vi "test222.vi"() -> ()   [LabVIEW 2014]
uses:
  ProjectLocker/NHMFL/LANL/Libraries/maglab ultrasound -- arkady/cursor winow.ctl
  ProjectLocker/NHMFL/LANL/Libraries/maglab ultrasound -- arkady/cursor window action.ctl
panel:
  in  "cursor bracket: All, data window":T1={"left"=3611.67564952785, "right "=3696.4045104721504, "center"=3654.04008, "window"=84.7288609443, "cursors"=[0, 1, 2], "relative"=1, "absolute"=1, "fixed vertical offset"=0.0, "vertical offset"=0.0, "skew"=0.0, "default window frac"=0.1, "kind"=enum."symmetric", "skew.left"=0.5, "skew.right"=0.5, "Plot ref"=refnum, "wing order"=enum."forw"}
  out "Plot: All":cluster{"all rows":dbl[], "all rows":dbl[]}[](graph)
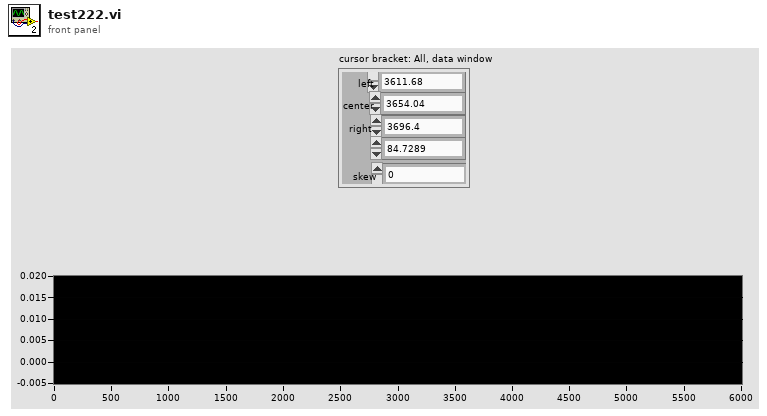
[diagram p1: front panel]
types:
  T1 = typedef "cursor winow.ctl" = cluster{"left":dbl, "right ":dbl, "center":dbl, "window":dbl, "cursors":i32[], "relative":i32, "absolute":i32, "fixed vertical offset":dbl, "vertical offset":dbl, "skew":dbl, "default window frac":dbl, "kind":enum16{"symmetric", "skewed", "fancy"}, "skew.left":dbl, "skew.right":dbl, "Plot ref":refnum<vi>, "wing order":enum16{"forw", "back"}}
  T2 = typedef "cursor window action.ctl" = enum16{"balance", "h. offset change", "cursor moves", "change center", "change window", "init", "check", "reset", "set y to middle", "idle", "-write all Y", "-write left.X", "-write center.X", "-write right.X", "-write all X", "-change center", "-change window", "-change skew", "-read cursor 2", "-read cursor 1", "-read cursor 0", "-read all cursors", "-reset", "-read plot scale", "-set y to middle", "-Q: center.Y is visible", "-Q: window is visible", "-parse center.Y", "-right left from center", "-left move", "-right move", "-set center.Y", "-empty", "-set cursors to default", "-check", "-write center.Y", "-copy cursor 1", "-copy cursor 0", "-copy cursor 2", "move right", "move left", "shrink", "broaden", "skew up", "skew down", "-write plot scale", "zoom X", "change cen&win", "zoom to all data"}
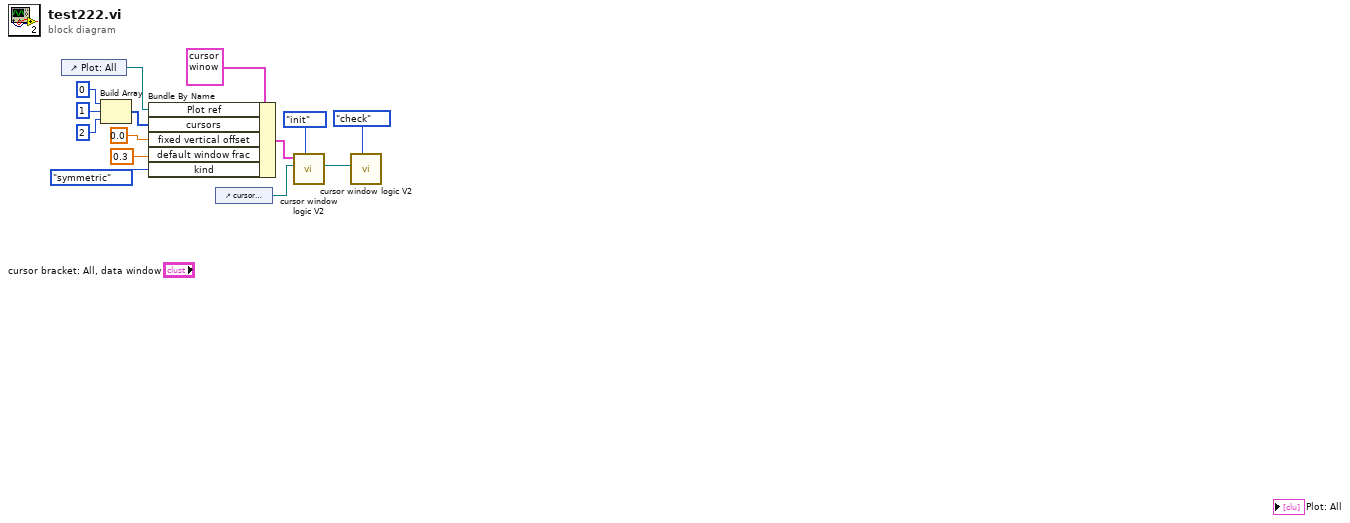
[diagram p0: block diagram]
diagram:
  n1 = control-ref of="Plot: All"() -> (w6:refnum<vi>)
  n2 = Build Array(0, 1, 2) -> (w14:i32[])
  n3 = Bundle By Name(cluster=T1 {"left"=0.0, "right "=0.0, "center"=0.0, "window"=0.0, "cursors"=[], "relative"=0, "absolute"=0, "fixed vertical offset"=0.0, "vertical offset"=0.0, "skew"=0.0, "default window frac"=0.0, "kind"=enum."symmetric", "skew.left"=0.0, "skew.right"=0.0, "Plot ref"=refnum, "wing order"=enum."forw"} ("cursor bracket: All, data window"), "Plot ref"=w6, "cursors"=w14, "fixed vertical offset"=0.0, "default window frac"=0.3 ("fixed vertical offset"), "kind"=enum16{"symmetric", "skewed", "fancy"}."symmetric") -> (w5:T1)
  n4 = control-ref of="cursor bracket: All, data window"() -> (w4:refnum<vi>)
  n5 = call "cursor window logic V2.vi"("cursor window action"=cursor_window_action."init", "cursor window in"=w4, "cursor window init"=w5) -> ("cursor window out"=w2:refnum<vi>)  [unwired: 7 in, 1 out]
  n6 = call "cursor window logic V2.vi"("cursor window action"=cursor_window_action."check", "cursor window in"=w2) -> ()  [unwired: 8 in, 2 out]
